vi "Get Attribute Visitor.vi"(8 "error in (no error)":errorcluster, 11 "NextGenXMLTypeGenerator in":refnum<class "NextGenXMLTypeGenerator.lvclass">) -> (0 "error out":errorcluster, 2 "Attribute Visitor":refnum<class "GetTypeAttributesVisitor.lvclass">, 3 "NextGenXMLTypeGenerator out":refnum<class "NextGenXMLTypeGenerator.lvclass">)   [LabVIEW 2020, in "Web Service Description.lvlib" / "NextGenXMLTypeGenerator.lvclass"]
uses:
  <vilib>/AppBuilder/Engine/WebServiceDescription/NextGenXMLTypeGenerator/NextGenXMLTypeGenerator.lvclass
  <vilib>/AppBuilder/Engine/WebServiceDescription/GetTypeAttributesVisitor/GetTypeAttributesVisitor.lvclass
  <vilib>/AppBuilder/Engine/WebServiceDescription/NextGenXMLTypeGenerator/NextGenXMLTypeGenerator.lvclass/NextGenXMLTypeGenerator.ctl
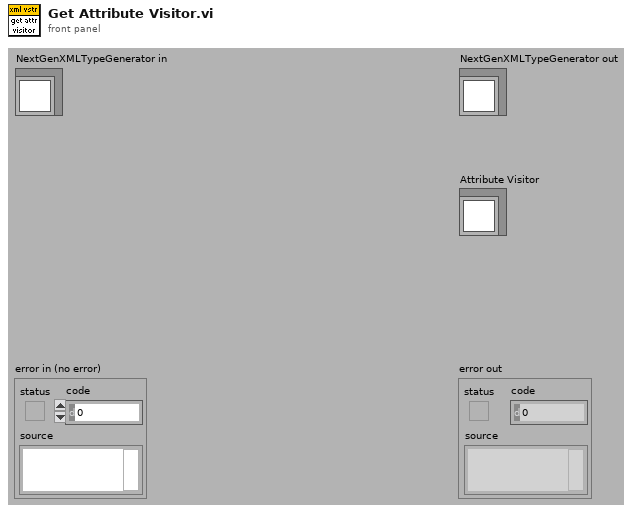
[diagram p1: front panel]
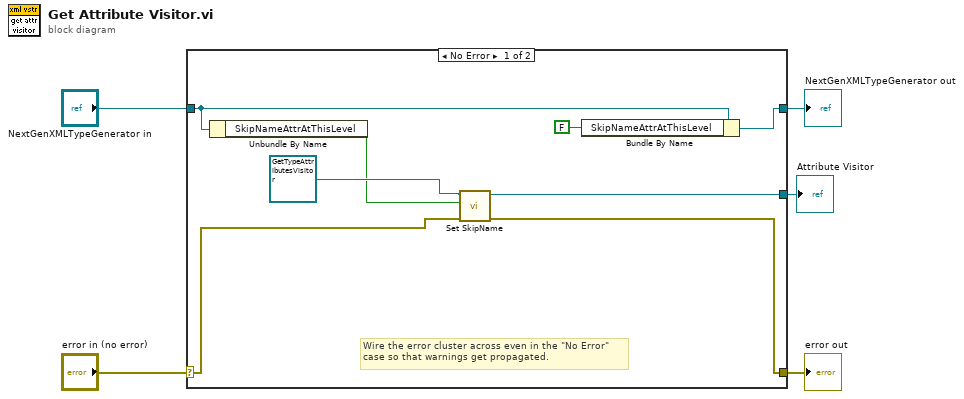
[diagram p0: block diagram]
diagram:
  n1 = case shown="No Error" "error in (no error)" {
    selector: "error in (no error)" -> [w12 w15]
    tunnel: [w6 w15] -> w4
    tunnel: [w10 w14] -> w2
    tunnel: "NextGenXMLTypeGenerator in" -> [w11 w14]
    tunnel: [w7 _] -> w1
    frame No Error {
      # "Wire the error cluster across even in the \"No Error\"\ncase so that warnings get propagated."
      n2 = Unbundle By Name(w11) -> ("SkipNameAttrAtThisLevel"=w9:bool)
      n3 = call <vilib>:"Set SkipName.vi"("error in (no error)"=w12, "SkipName"=w9, "GetTypeAttributesVisitor.lvclass in"=refnum<class "GetTypeAttributesVisitor.lvclass"> refnum ("Web Service Description.lvlib:GetTypeAttributesVisitor.lvclass")) -> ("error out"=w6:errorcluster, "GetTypeAttributesVisitor.lvclass out"=w7:refnum<class "GetTypeAttributesVisitor.lvclass">)  [unwired: 7 out]
      n4 = Bundle By Name(cluster=w11, "SkipNameAttrAtThisLevel"=FALSE) -> (w10:refnum<class "NextGenXMLTypeGenerator.lvclass">)
    }
    frame Error {
    }
  }
  "error out" <- w4
  "NextGenXMLTypeGenerator out" <- w2
  "Attribute Visitor" <- w1
